vi "Generate Value.vi"(6 "time stamp":timestamp, 8 "error in (no error)":errorcluster, 10 "base value":i64, 11 "value in":refnum<class "NT Base.lvclass">) -> (0 "error out":errorcluster, 3 "value out":refnum<class "NT Base.lvclass">)   [LabVIEW 2020]
uses:
  source/PV Data/NT Base/NT Base.lvclass
  source/PV Data/NT Scalar/NT Scalar.lvclass
  C:/Users/eyw68381/source/repos/pvaccess-labview/labview/source/PV Data/NT Base/NT Base.lvclass
  source/PV Data/NT Enum/NT Enum.lvclass
  3336d5e6-6b46-40cc-8581-c00a96048cf3.vi
  c0315305-4ea9-43e2-99a8-a5923f228944.vi
  e9ef65dd-4b85-465f-aa80-4b18505edb13.vi
  babcc117-bc44-41a1-9c2b-73189d1bbfcb.vi
  c68d18eb-9334-419f-972f-f5b5be29402e.vi
  54e220c7-dbf9-4865-aabc-812fe05ebb8b.vi
  47823474-13c3-4f35-a55b-4dd444e3f7d9.vi
  e6de0aaa-8fd3-4213-bbd6-031fb177ed83.vi
  115dbf5b-fdea-438f-8eda-7315cadb6382.vi
  228aee6f-7479-4422-86e8-739061133d5f.vi
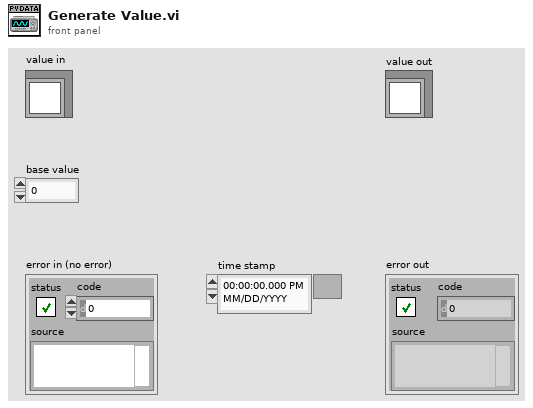
[diagram p1: front panel]
types:
  T1 = typedef "PV Access.lvlib/PV Data.lvlib/Type Code.ctl" = enum8{"Null", "Bool", "BoolA", "Int8", "Int8A", "Int16", "Int16A", "Int32", "Int32A", "Int64", "Int64A", "UInt8", "UInt8A", "UInt16", "UInt16A", "UInt32", "UInt32A", "UInt64", "UInt64A", "Float32", "Float32A", "Float64", "Float64A", "String", "StringA", "Struct", "StructA", "Union", "UnionA", "Any", "AnyA"}
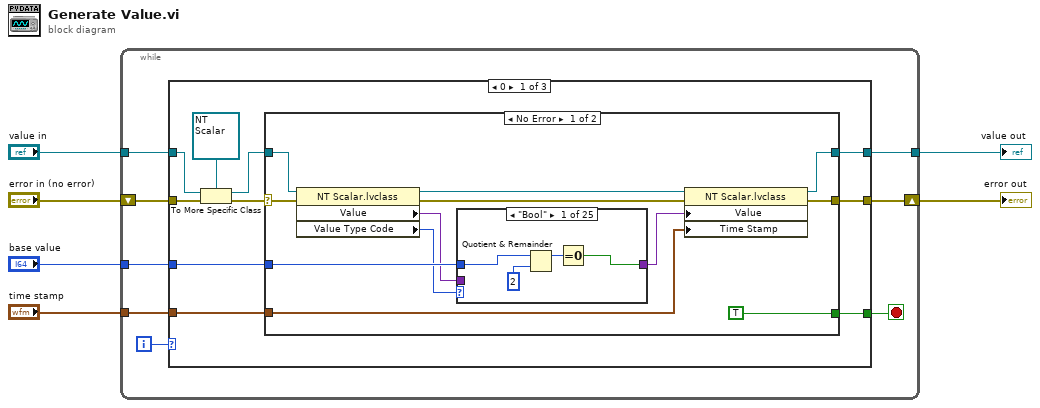
[diagram p0: block diagram]
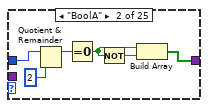
[diagram p2: hidden frame]
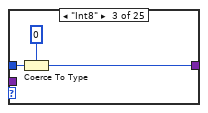
[diagram p3: hidden frame]
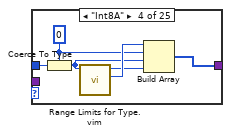
[diagram p4: hidden frame]
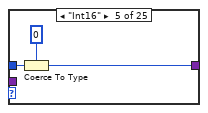
[diagram p5: hidden frame]
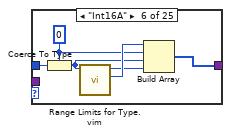
[diagram p6: hidden frame]
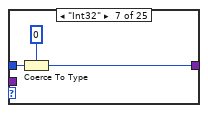
[diagram p7: hidden frame]
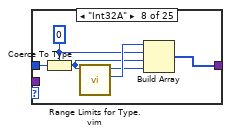
[diagram p8: hidden frame]
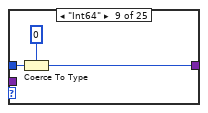
[diagram p9: hidden frame]
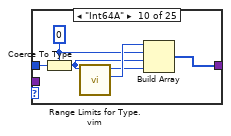
[diagram p10: hidden frame]
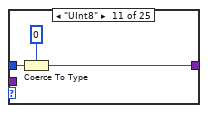
[diagram p11: hidden frame]
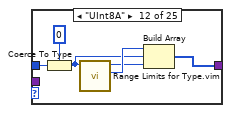
[diagram p12: hidden frame]
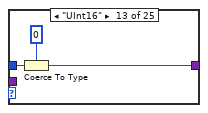
[diagram p13: hidden frame]
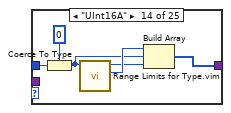
[diagram p14: hidden frame]
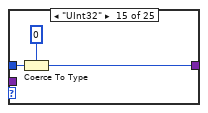
[diagram p15: hidden frame]
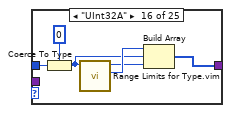
[diagram p16: hidden frame]
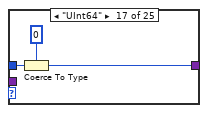
[diagram p17: hidden frame]
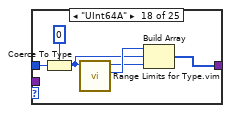
[diagram p18: hidden frame]
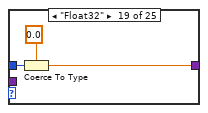
[diagram p19: hidden frame]
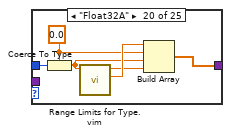
[diagram p20: hidden frame]
diagram:
  n1 = while {
    tunnel: "base value" -> [w14]
    tunnel: [w13] -> w5
    tunnel: "value in" -> [w10]
    shift-right: [w11] -> w3
    shift-left: "error in (no error)" -> [w12]
    tunnel: "time stamp" -> [w7]
    i -> [w9]
    stop <- w8 stop-if-true
    n2 = case shown="0" w9 {
      tunnel: w14 -> [w24 w156 _]
      tunnel: [w23 w155 w174] -> w13
      tunnel: w12 -> [w17 w149 w173]
      tunnel: [w22 w154 w173] -> w11
      tunnel: w10 -> [w21 w153 w174]
      tunnel: [w16 w148 TRUE] -> w8
      tunnel: w7 -> [w15 _ _]
      frame 0 {
        n3 = To More Specific Class(target class=refnum<class "NT Scalar.lvclass"> refnum ("PV Access.lvlib:PV Data.lvlib:NT Scalar.lvclass"), reference=w21, error in=w17) -> (specific class reference=w18:refnum<class "NT Scalar.lvclass">, error out=w19:errorcluster)
        n4 = case shown="No Error" w19 {
          selector: w19 -> [w35 w146]
          tunnel: w24 -> [w36 _]
          tunnel: [w27 w147] -> w23
          tunnel: [w28 w145] -> w22
          tunnel: w18 -> [w34 w147]
          tunnel: [TRUE _] -> w16
          tunnel: w15 -> [w25 _]
          frame No Error {
            n5 = property class="NT Scalar.lvclass"(reference=w34, error in=w35) -> (reference out=w30:refnum<class "NT Scalar.lvclass">, error out=w31:errorcluster, "Value"=w32:variant, "Value Type Code"=w33:T1)
            n6 = case shown="\"Bool\"" w33 {
              tunnel: w36 -> [w39 w44 w48 w55 w57 w64 w66 w73 w75 w82 w84 w91 w93 w100 w102 w109 w111 w118 w120 w127 w129 w136 w138 w142 _]
              tunnel: [w38 w46 w47 w54 w56 w63 w65 w72 w74 w81 w83 w90 w92 w99 w101 w108 w110 w117 w119 w126 w128 w135 w137 w139 w143] -> w29
              tunnel: w32 -> [_ _ _ _ _ _ _ _ _ _ _ _ _ _ _ _ _ _ _ _ _ _ _ _ w143]
              frame "Bool" {
                n7 = Quotient & Remainder(x=w39, y=i64 2) -> (x-y*floor(x/y)=w37:i64)  [unwired: 1 out]
                n8 = Equal To 0?(x=w37) -> (x = 0?=w38:bool)
              }
              frame "BoolA" {
                n9 = Quotient & Remainder(x=w44, y=i64 2) -> (x-y*floor(x/y)=w43:i64)  [unwired: 1 out]
                n10 = Equal To 0?(x=w43) -> (x = 0?=w41:bool)
                n11 = Not(x=w41) -> (.not. x?=w42:bool)
                n12 = Build Array(w41, w42) -> (w46:bool[])
              }
              frame "Int8" {
                n13 = Coerce To Type(0:w48, 1:i8 0 ("default value")) -> (2:w47:i8)
              }
              frame "Int8A" {
                w51 = i8 0 ("default value")
                n14 = Coerce To Type(0:w55, 1:w51) -> (2:w50:i8)
                n15 = call "Range Limits for Type.vim"("type"=w50) -> ("minimum value for type"=w53:i8, "maximum value for type"=w52:i8)  [unwired: 9 in]
                n16 = Build Array(w53, w51, w50, w52) -> (w54:i8[])
              }
              frame "Int16" {
                n17 = Coerce To Type(0:w57, 1:i16 0 ("default value")) -> (2:w56:i16)
              }
              frame "Int16A" {
                w60 = i16 0 ("default value")
                n18 = Coerce To Type(0:w64, 1:w60) -> (2:w59:i16)
                n19 = call "Range Limits for Type.vim"("type"=w59) -> ("minimum value for type"=w62:i16, "maximum value for type"=w61:i16)  [unwired: 9 in]
                n20 = Build Array(w62, w60, w59, w61) -> (w63:i16[])
              }
              frame "Int32" {
                n21 = Coerce To Type(0:w66, 1:0 ("default value")) -> (2:w65:i32)
              }
              frame "Int32A" {
                w69 = 0 ("default value")
                n22 = Coerce To Type(0:w73, 1:w69) -> (2:w68:i32)
                n23 = call "Range Limits for Type.vim"("type"=w68) -> ("minimum value for type"=w71:i32, "maximum value for type"=w70:i32)  [unwired: 9 in]
                n24 = Build Array(w71, w69, w68, w70) -> (w72:i32[])
              }
              frame "Int64" {
                n25 = Coerce To Type(0:w75, 1:i64 0 ("default value")) -> (2:w74:i64)
              }
              frame "Int64A" {
                w78 = i64 0 ("default value")
                n26 = Coerce To Type(0:w82, 1:w78) -> (2:w77:i64)
                n27 = call "Range Limits for Type.vim"("type"=w77) -> ("minimum value for type"=w80:i64, "maximum value for type"=w79:i64)  [unwired: 9 in]
                n28 = Build Array(w80, w78, w77, w79) -> (w81:i64[])
              }
              frame "UInt8" {
                n29 = Coerce To Type(0:w84, 1:u8 0 ("default value")) -> (2:w83:u8)
              }
              frame "UInt8A" {
                n30 = Coerce To Type(0:w91, 1:u8 0 ("default value")) -> (2:w87:u8)
                n31 = call "Range Limits for Type.vim"("type"=w87) -> ("minimum value for type"=w89:u8, "maximum value for type"=w86:u8)  [unwired: 9 in]
                n32 = Build Array(w89, w87, w86) -> (w90:u8[])
              }
              frame "UInt16" {
                n33 = Coerce To Type(0:w93, 1:u16 0 ("default value")) -> (2:w92:u16)
              }
              frame "UInt16A" {
                n34 = Coerce To Type(0:w100, 1:u16 0 ("default value")) -> (2:w96:u16)
                n35 = call "Range Limits for Type.vim"("type"=w96) -> ("minimum value for type"=w98:u16, "maximum value for type"=w95:u16)  [unwired: 9 in]
                n36 = Build Array(w98, w96, w95) -> (w99:u16[])
              }
              frame "UInt32" {
                n37 = Coerce To Type(0:w102, 1:u32 0 ("default value")) -> (2:w101:u32)
              }
              frame "UInt32A" {
                n38 = Coerce To Type(0:w109, 1:u32 0 ("default value")) -> (2:w105:u32)
                n39 = call "Range Limits for Type.vim"("type"=w105) -> ("minimum value for type"=w107:u32, "maximum value for type"=w104:u32)  [unwired: 9 in]
                n40 = Build Array(w107, w105, w104) -> (w108:u32[])
              }
              frame "UInt64" {
                n41 = Coerce To Type(0:w111, 1:u64 0 ("default value")) -> (2:w110:u64)
              }
              frame "UInt64A" {
                n42 = Coerce To Type(0:w118, 1:u64 0 ("default value")) -> (2:w114:u64)
                n43 = call "Range Limits for Type.vim"("type"=w114) -> ("minimum value for type"=w116:u64, "maximum value for type"=w113:u64)  [unwired: 9 in]
                n44 = Build Array(w116, w114, w113) -> (w117:u64[])
              }
              frame "Float32" {
                n45 = Coerce To Type(0:w120, 1:sgl 0.0 ("default value")) -> (2:w119:sgl)
              }
              frame "Float32A" {
                w123 = sgl 0.0 ("default value")
                n46 = Coerce To Type(0:w127, 1:w123) -> (2:w122:sgl)
                n47 = call "Range Limits for Type.vim"("type"=w122) -> ("minimum value for type"=w125:sgl, "maximum value for type"=w124:sgl)  [unwired: 9 in]
                n48 = Build Array(w125, w123, w122, w124) -> (w126:sgl[])
              }
              frame "Float64" {
                n49 = Coerce To Type(0:w129, 1:0.0 ("default value")) -> (2:w128:dbl)
              }
              frame "Float64A" {
                w132 = 0.0 ("default value")
                n50 = Coerce To Type(0:w136, 1:w132) -> (2:w131:dbl)
                n51 = call "Range Limits for Type.vim"("type"=w131) -> ("minimum value for type"=w134:dbl, "maximum value for type"=w133:dbl)  [unwired: 9 in]
                n52 = Build Array(w134, w132, w131, w133) -> (w135:dbl[])
              }
              frame "String" {
                n53 = Format Value(value (0)=w138) -> (output string=w137:string)  [unwired: 2 in]
              }
              frame "StringA" {
                n54 = Format Value(value (0)=w142) -> (output string=w141:string)  [unwired: 2 in]
                n55 = Build Array(w141, "Hello" ("element")) -> (w139:string[])
              }
              frame Default {
              }
            }
            n56 = property class="NT Scalar.lvclass"(reference=w30, error in=w31, "Value"=w29, "Time Stamp"=w25) -> (reference out=w27:refnum<class "NT Scalar.lvclass">, error out=w28:errorcluster)
          }
          frame Error {
            n57 = call <vilib>:"Clear Errors.vi"("error in (no error)"=w146, "specific error code to clear (0: all)"=1448) -> ("error out"=w145:errorcluster)  [unwired: 4 in, 1 out]
          }
        }
      }
      frame 1 {
        n58 = To More Specific Class(target class=refnum<class "NT Enum.lvclass"> refnum ("PV Access.lvlib:PV Data.lvlib:NT Enum.lvclass"), reference=w153, error in=w149) -> (specific class reference=w150:refnum<class "NT Enum.lvclass">, error out=w151:errorcluster)
        n59 = case shown="Error .." w151 {
          selector: w151 -> [w167 w170]
          tunnel: w156 -> [w158 _]
          tunnel: [w162 w171] -> w155
          tunnel: [w163 w169] -> w154
          tunnel: w150 -> [w166 w171]
          tunnel: [TRUE _] -> w148
          frame No Error {
            n60 = property class="NT Enum.lvclass"(reference=w166, error in=w167) -> (reference out=w164:refnum<class "NT Enum.lvclass">, error out=w165:errorcluster, "Choices"=w160:string[])
            n61 = Array Size(array=w160) -> (size(s)=w159:i32)
            n62 = Quotient & Remainder(x=w158, y=w159) -> (x-y*floor(x/y)=w157:i64)  [unwired: 1 out]
            n63 = property class="NT Enum.lvclass"(reference=w164, error in=w165, "Index"=w157) -> (reference out=w162:refnum<class "NT Enum.lvclass">, error out=w163:errorcluster)
          }
          frame Error {
            n64 = call <vilib>:"Clear Errors.vi"("error in (no error)"=w170, "specific error code to clear (0: all)"=1448) -> ("error out"=w169:errorcluster)  [unwired: 4 in, 1 out]
          }
        }
      }
      frame Default {
      }
    }
  }
  "value out" <- w5
  "error out" <- w3
